vi "run.update_commit.vi"(8 "error in":errorcluster, 11 "RunUpdateStaging in":refnum<class "RunUpdateStaging.lvclass">) -> (0 "error out":errorcluster, 3 "RunUpdateStaging out":refnum<class "RunUpdateStaging.lvclass">)   [LabVIEW 2020, in "RunUpdateStaging.lvclass"]
doc: "Applies the staged changes to the run and returns a handle to the updated run."
uses:
  RunUpdateStaging.lvclass
  RunUpdateStaging.lvclass/RunUpdateStaging.ctl
  client.lvlib
panel:
  out "out_run out":i32
  in  "rid":string
  in  "staging":i32
  in  "out_run":i32
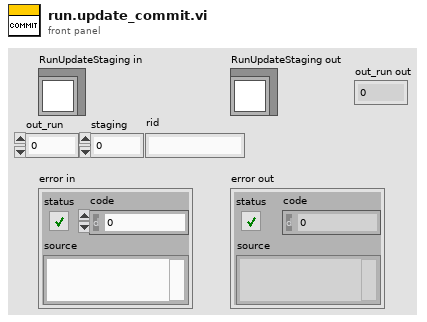
[diagram p1: front panel]
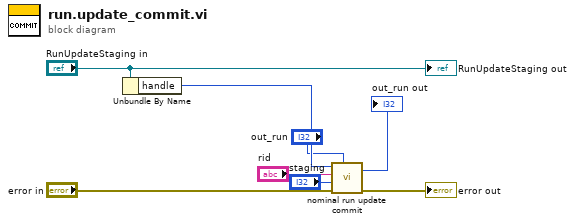
[diagram p0: block diagram]
diagram:
  n1 = Unbundle By Name("RunUpdateStaging in") -> ("handle"=w6:i32)
  n2 = call "nominal run update commit.vi"("out_run"="out_run", "error in (no error)"="error in", "staging"="staging", "rid"="rid", "client"=w6) -> ("error out"=→"error out":errorcluster, "out_run out"=→"out_run out":i32)  [unwired: 4 in, 1 out]
  "RunUpdateStaging out" <- "RunUpdateStaging in"
